vi "AES DataReplay Calculate Voltage Scaler.vi"(8 "maximum voltage":dbl, 9 "maximum speed (RPM)":dbl, 10 "threshold voltage":dbl, 11 "threshold speed (RPM)":dbl) -> (2 "intercept (b)":fxp<+/-,18,3>, 3 "slope (m)":fxp<+,18,12>)   [LabVIEW 2010, in "AES.lvlib" / "AES RT.lvlib"]
doc: "This VI takes the configuration parameters for voltage scaling and calculates the slope and intercept (for y=mx+b) of the data replay voltage. The slope (m) and intercept (b) should then be sent to the FPGA for scaling data replay voltage."
uses:
  AES RT.lvlib
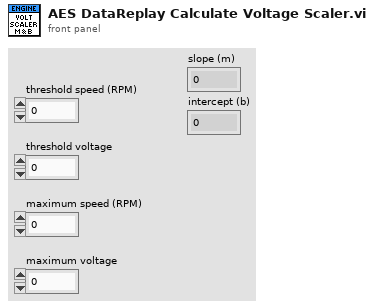
[diagram p1: front panel]
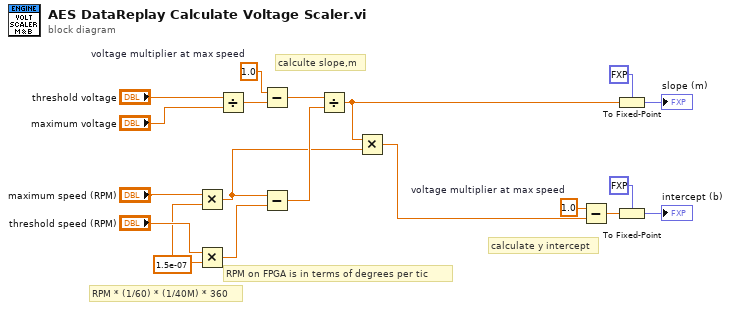
[diagram p0: block diagram]
diagram:
  w4 = 1.5e-07 ("y")
  w13 = 1.0  # voltage multiplier at max speed
  w16 = 1.0  # voltage multiplier at max speed
  # "RPM * (1/60) * (1/40M) * 360"
  # "RPM on FPGA is in terms of degrees per tic"
  # "calculate y intercept"
  # "calculte slope,m"
  n1 = Multiply(x="maximum speed (RPM)", y=w4) -> (x*y=w3:dbl)
  n2 = Multiply(x="threshold speed (RPM)", y=w4) -> (x*y=w6:dbl)
  n3 = Divide(x="threshold voltage", y="maximum voltage") -> (x/y=w17:dbl)
  n4 = Subtract(x=w16, y=w17) -> (x-y=w15:dbl)
  n5 = Subtract(x=w3, y=w6) -> (x-y=w14:dbl)
  n6 = Divide(x=w15, y=w14) -> (x/y=w9:dbl)
  n7 = Multiply(x=w9, y=w3) -> (x*y=w12:dbl)
  n8 = Subtract(x=w13, y=w12) -> (x-y=w8:dbl)
  n9 = To Fixed-Point(fixed-point type=fxp<+,18,12> 0.0, number=w9) -> (fixed-point=→"slope (m)":fxp<+,18,12>)
  n10 = To Fixed-Point(fixed-point type=fxp<+/-,18,3> 0.0, number=w8) -> (fixed-point=→"intercept (b)":fxp<+/-,18,3>)
